vi "Result_Array_manipulation.vi"(8 "Array of Overlay Lines":T5(array[cluster]), 9 "SplitCameraID":i32[](array[numeric]), 10 "Camera ID":i32[](array[numeric]), 11 "Result Cluster":T1={"Measurement Names Array"=[], "Pass-Fail Array"=[], "Measurement Values Array "=[], "Roi for overlay (Arrows) Array"=[], "Algo Type Array"=[], "Image Array"=[], "Clamp operations"=enum."Average Clamp", "  Search Direction "=[], "Images_Array_in"=[], "ResultPF"=FALSE, "Total Cluster Values"={"Total Fail"=0, "Total Pass"=0, "Total Count"=0}, "Reel Counter Cluster"={"Reel Fail"=0, "Reel Pass"=0, "Reel Count"=0}, "Tolerance  Array"=[], "Array of Cam Spec Control Bool"=[], "Control Pass Fail Array"=[], "Specification Pass Fail Array"=[], "Overlay Arrow Lines"=[], "Camera ID"=[], "Trigger count"=0, "Specification fail?"=FALSE}) -> (2 "Result_Cam_2":T4, 3 "Result_Cam_0_1":T3)   [LabVIEW 2019, in "Algorithm.lvclass"]
uses:
  FrameworkOverrides/Algorithm.lvclass
  <vilib>/vision/Image Controls.llb/IMAQ Image.ctl
  Controls/Result Cluster.ctl
panel:
  out "Array 3":i32[](array[numeric])
  out "CamID_0_1":T2[](array[typedef])
  out "CamID_2":T2[](array[typedef])
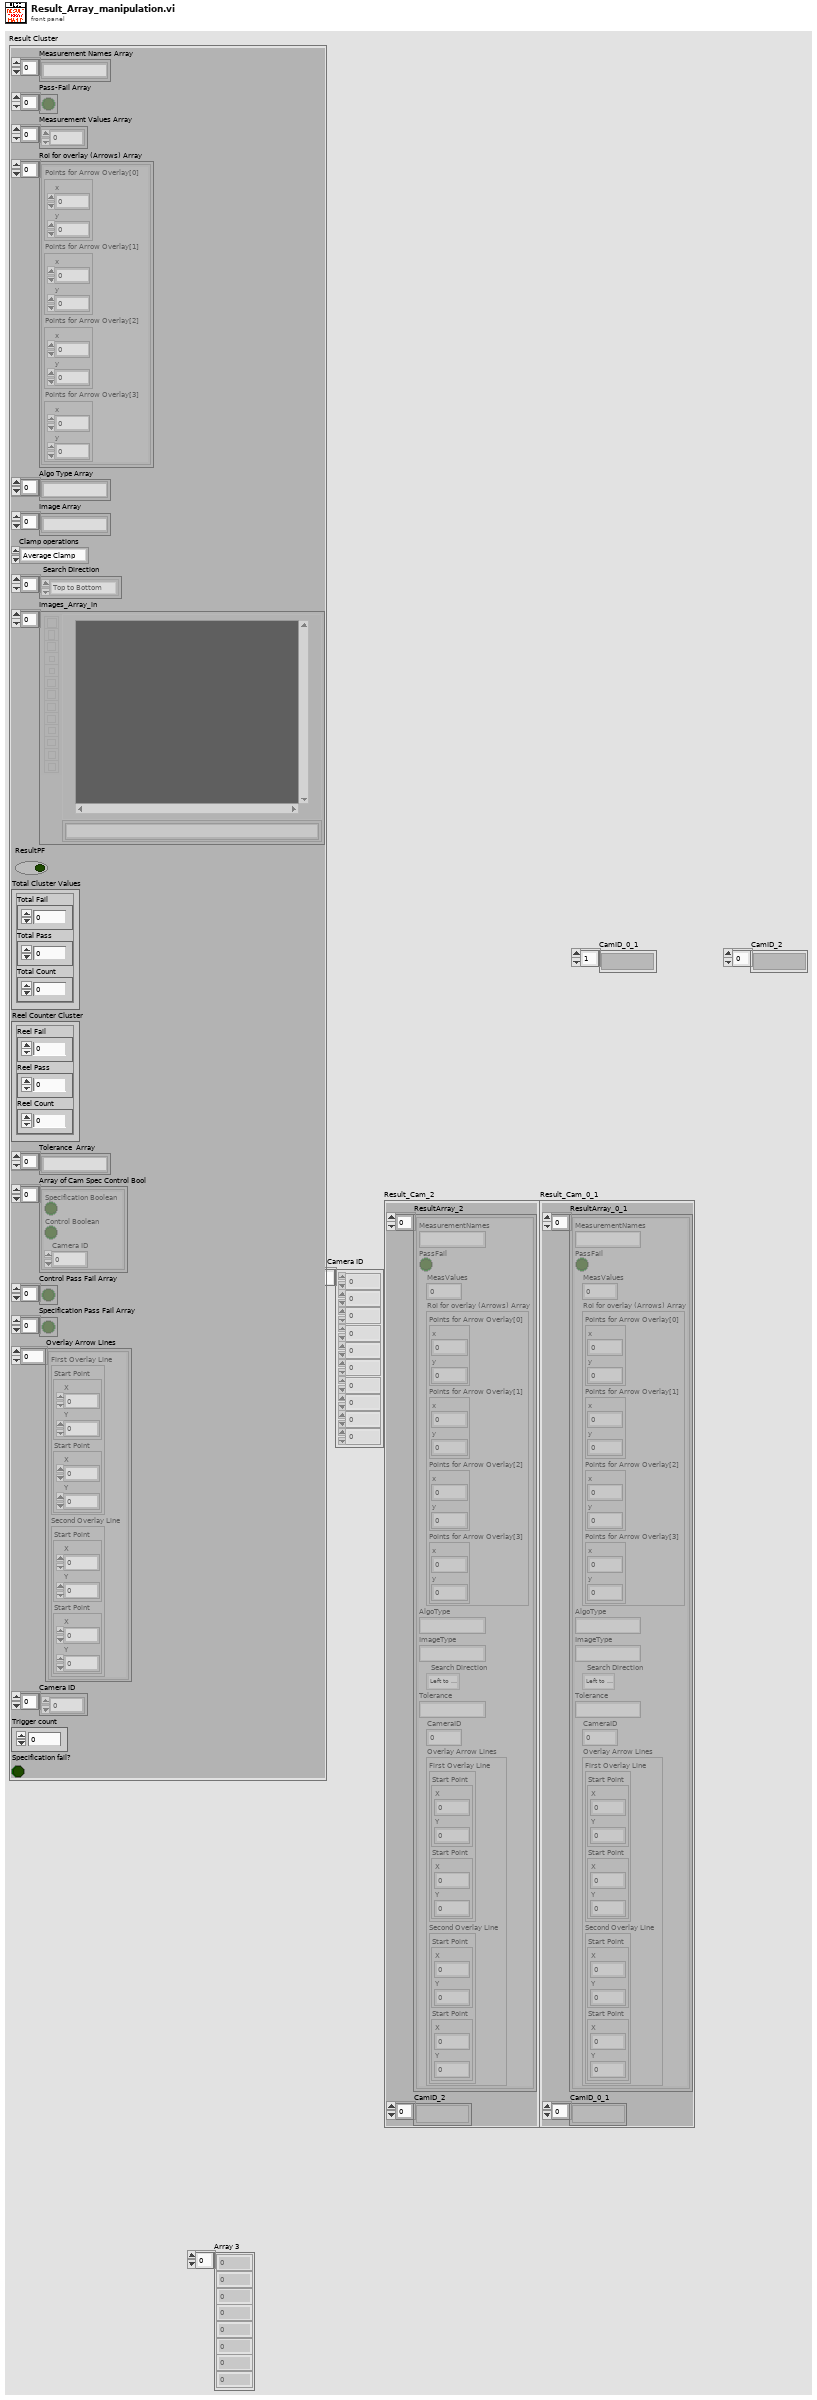
[diagram p1: front panel]
types:
  T1 = typedef "Algorithm.lvclass/Result Cluster.ctl" = cluster{"Measurement Names Array":string[], "Pass-Fail Array":bool[], "Measurement Values Array ":dbl[], "Roi for overlay (Arrows) Array":cluster{"Points for Arrow Overlay[0]":cluster{"x":dbl, "y":dbl}, "Points for Arrow Overlay[1]":cluster{"x":dbl, "y":dbl}, "Points for Arrow Overlay[2]":cluster{"x":dbl, "y":dbl}, "Points for Arrow Overlay[3]":cluster{"x":dbl, "y":dbl}}[], "Algo Type Array":string[], "Image Array":string[], "Clamp operations":enum16{"Min Clamp", "Max Clamp", "Average Clamp"}, "  Search Direction ":enum16{"Left to Right", "Right to Left", "Top to Bottom", "Bottom to Top"}[], "Images_Array_in":T2[], "ResultPF":bool, "Total Cluster Values":cluster{"Total Fail":u64, "Total Pass":u64, "Total Count":u64}, "Reel Counter Cluster":cluster{"Reel Fail":u64, "Reel Pass":u64, "Reel Count":u64}, "Tolerance  Array":string[], "Array of Cam Spec Control Bool":cluster{"Specification Boolean":bool, "Control Boolean":bool, "Camera ID":i8}[], "Control Pass Fail Array":bool[], "Specification Pass Fail Array":bool[], "Overlay Arrow Lines":cluster{"First Overlay Line ":cluster{"Start Point":cluster{"X":sgl, "Y":sgl}, "Start Point":cluster{"X":sgl, "Y":sgl}}, "Second Overlay Line ":cluster{"Start Point":cluster{"X":sgl, "Y":sgl}, "Start Point":cluster{"X":sgl, "Y":sgl}}}[], "Camera ID":i8[], "Trigger count":i32, "Specification fail?":bool}
  T2 = typedef "IMAQ Image.ctl" = refnum<image>
  T3 = cluster{"ResultArray_0_1":cluster{"MeasurementNames":string, "PassFail":bool, "MeasValues":dbl, "Roi for overlay (Arrows) Array":cluster{"Points for Arrow Overlay[0]":cluster{"x":dbl, "y":dbl}, "Points for Arrow Overlay[1]":cluster{"x":dbl, "y":dbl}, "Points for Arrow Overlay[2]":cluster{"x":dbl, "y":dbl}, "Points for Arrow Overlay[3]":cluster{"x":dbl, "y":dbl}}, "AlgoType":string, "ImageType":string, "  Search Direction ":enum16{"Left to Right", "Right to Left", "Top to Bottom", "Bottom to Top"}, "Tolerance":string, "CameraID":i32, "Overlay Arrow Lines":cluster{"First Overlay Line ":cluster{"Start Point":cluster{"X":sgl, "Y":sgl}, "Start Point":cluster{"X":sgl, "Y":sgl}}, "Second Overlay Line ":cluster{"Start Point":cluster{"X":sgl, "Y":sgl}, "Start Point":cluster{"X":sgl, "Y":sgl}}}}[], "CamID_0_1":T2[]}
  T4 = cluster{"ResultArray_2":cluster{"MeasurementNames":string, "PassFail":bool, "MeasValues":dbl, "Roi for overlay (Arrows) Array":cluster{"Points for Arrow Overlay[0]":cluster{"x":dbl, "y":dbl}, "Points for Arrow Overlay[1]":cluster{"x":dbl, "y":dbl}, "Points for Arrow Overlay[2]":cluster{"x":dbl, "y":dbl}, "Points for Arrow Overlay[3]":cluster{"x":dbl, "y":dbl}}, "AlgoType":string, "ImageType":string, "  Search Direction ":enum16{"Left to Right", "Right to Left", "Top to Bottom", "Bottom to Top"}, "Tolerance":string, "CameraID":i32, "Overlay Arrow Lines":cluster{"First Overlay Line ":cluster{"Start Point":cluster{"X":sgl, "Y":sgl}, "Start Point":cluster{"X":sgl, "Y":sgl}}, "Second Overlay Line ":cluster{"Start Point":cluster{"X":sgl, "Y":sgl}, "Start Point":cluster{"X":sgl, "Y":sgl}}}}[], "CamID_2":T2[]}
  T5 = cluster{"First Overlay Line ":cluster{"Start Point":cluster{"X":sgl, "Y":sgl}, "Start Point":cluster{"X":sgl, "Y":sgl}}, "Second Overlay Line ":cluster{"Start Point":cluster{"X":sgl, "Y":sgl}, "Start Point":cluster{"X":sgl, "Y":sgl}}}[]
  T6 = cluster{"MeasurementNames":string, "PassFail":bool, "MeasValues":dbl, "Roi for overlay (Arrows) Array":cluster{"Points for Arrow Overlay[0]":cluster{"x":dbl, "y":dbl}, "Points for Arrow Overlay[1]":cluster{"x":dbl, "y":dbl}, "Points for Arrow Overlay[2]":cluster{"x":dbl, "y":dbl}, "Points for Arrow Overlay[3]":cluster{"x":dbl, "y":dbl}}, "AlgoType":string, "ImageType":string, "  Search Direction ":enum16{"Left to Right", "Right to Left", "Top to Bottom", "Bottom to Top"}, "Tolerance":string, "CameraID":i32, "Overlay Arrow Lines":cluster{"First Overlay Line ":cluster{"Start Point":cluster{"X":sgl, "Y":sgl}, "Start Point":cluster{"X":sgl, "Y":sgl}}, "Second Overlay Line ":cluster{"Start Point":cluster{"X":sgl, "Y":sgl}, "Start Point":cluster{"X":sgl, "Y":sgl}}}}
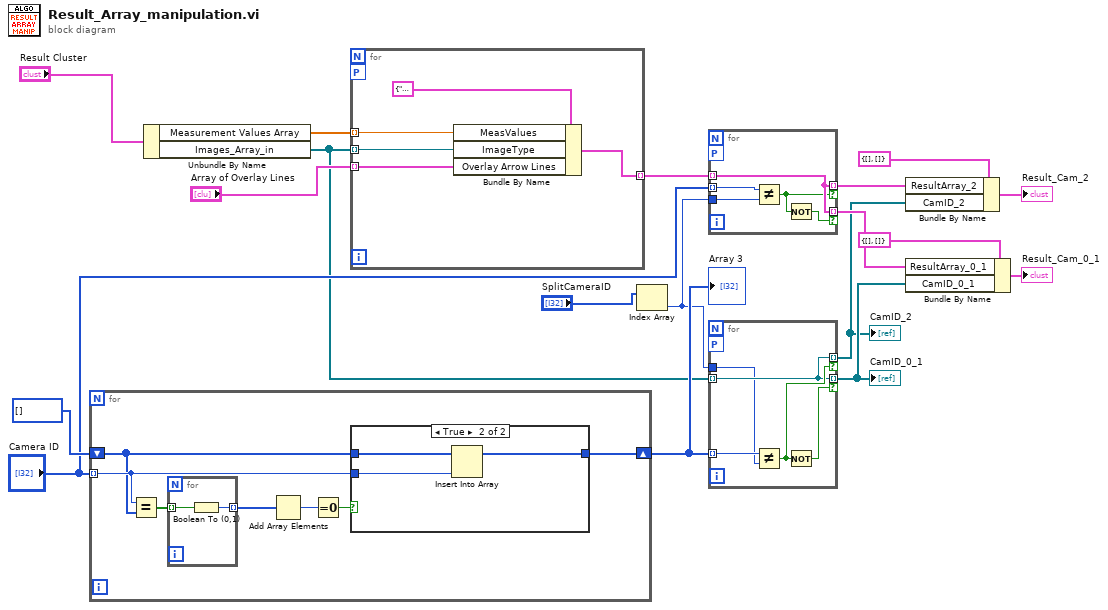
[diagram p0: block diagram]
diagram:
  n1 = for {
    tunnel: "Camera ID" -> [w24] mode=indexing
    shift-right: [w25] -> w13
    shift-left: i32[] [] -> [w23]
    n2 = Equal?(x=w24, y=w23) -> (x = y?=w22:bool[])
    n3 = for {
      tunnel: w22 -> [w27] mode=indexing
      tunnel: [w26] -> w21 mode=indexing
      n4 = Boolean To (0,1)(Boolean=w27) -> (0, 1=w26:i16)
    }
    n5 = Add Array Elements(numeric array=w21) -> (sum=w20:i16)
    n6 = Equal To 0?(x=w20) -> (x = 0?=w19:bool)
    n7 = case shown="True" w19 {
      tunnel: w24 -> [_ w31]
      tunnel: [w28 w30] -> w25
      tunnel: w23 -> [w28 w29]
      frame False {
      }
      frame True {
        n8 = Insert Into Array(array=w29, new element=w31) -> (w30:i32[])  [unwired: 1 in]
      }
    }
  }
  "Array 3" <- w13
  n9 = Unbundle By Name("Result Cluster") -> ("Measurement Values Array"=w18:dbl[], "Images_Array_in"=w2:T2[])
  n10 = for {
    tunnel: w18 -> [w36] mode=indexing
    tunnel: w2 -> [w35] mode=indexing
    tunnel: [w34] -> w17 mode=indexing
    workers-P: _ -> [_]
    tunnel: "Array of Overlay Lines" -> [w32] mode=indexing
    n11 = Bundle By Name(cluster=T6 {"MeasurementNames"="", "PassFail"=TRUE, "MeasValues"=0.0, "Roi for overlay (Arrows) Array"={"Points for Arrow Overlay[0]"={"x"=0.0, "y"=0.0}, "Points for Arrow Overlay[1]"={"x"=0.0, "y"=0.0}, "Points for Arrow Overlay[2]"={"x"=0.0, "y"=0.0}, "Points for Arrow Overlay[3]"={"x"=0.0, "y"=0.0}}, "AlgoType"="", "ImageType"="", "  Search Direction "=enum."Left to Right", "Tolerance"="", "CameraID"=0, "Overlay Arrow Lines"={"First Overlay Line "={"Start Point"={"X"=0.0, "Y"=0.0}, "Start Point"={"X"=0.0, "Y"=0.0}}, "Second Overlay Line "={"Start Point"={"X"=0.0, "Y"=0.0}, "Start Point"={"X"=0.0, "Y"=0.0}}}}, "MeasValues"=w36, "ImageType"=w35, "Overlay Arrow Lines"=w32) -> (w34:T6)
  }
  n12 = Index Array(array="SplitCameraID") -> (element=w7:i32)  [unwired: 1 in]
  n13 = for {
    tunnel: w17 -> [w41] mode=indexing
    tunnel: [w41] -> w6 mode=indexing if=w39
    tunnel: [w41] -> w16 mode=indexing if=w38
    tunnel: "Camera ID" -> [w40] mode=indexing
    tunnel: w7 -> [w37]
    workers-P: _ -> [_]
    n14 = Not Equal?(x=w40, y=w37) -> (x != y?=w39:bool)
    n15 = Not(x=w39) -> (.not. x?=w38:bool)
  }
  n16 = for {
    tunnel: w13 -> [w46] mode=indexing
    tunnel: w2 -> [w44] mode=indexing
    tunnel: [w44] -> w9 mode=indexing if=w45
    tunnel: [w44] -> w10 mode=indexing if=w43
    tunnel: w7 -> [w42]
    workers-P: _ -> [_]
    n17 = Not Equal?(x=w46, y=w42) -> (x != y?=w45:bool)
    n18 = Not(x=w45) -> (.not. x?=w43:bool)
  }
  "CamID_0_1" <- w10
  "CamID_2" <- w9
  n19 = Bundle By Name(cluster=T4 {"ResultArray_2"=[], "CamID_2"=[]}, "ResultArray_2"=w6, "CamID_2"=w9) -> (→"Result_Cam_2":T4)
  n20 = Bundle By Name(cluster=T3 {"ResultArray_0_1"=[], "CamID_0_1"=[]}, "ResultArray_0_1"=w16, "CamID_0_1"=w10) -> (→"Result_Cam_0_1":T3)
